vi "Write iterator.vi"(10 "iterator":refnum<data-value>, 11 "Circular Buffer in":refnum<class "Circular Buffer.lvclass">) -> (3 "Circular Buffer out":refnum<class "Circular Buffer.lvclass">)   [LabVIEW 2021, in "d20.lvlib" / "Circular Buffer.lvclass"]
uses:
  Circular Buffer.lvclass
  INode/INode.lvclass
  Circular Buffer.lvclass/Circular Buffer.ctl
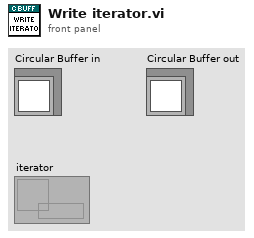
[diagram p1: front panel]
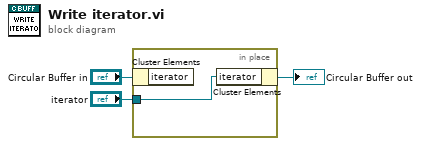
[diagram p0: block diagram]
diagram:
  n1 = in-place {
    in-place-border: "iterator" -> [w4]
    n2 = in-place-cluster #1("Circular Buffer in") -> ()  [unwired: 1 out]
    n3 = in-place-cluster #1("iterator"=w4) -> (→"Circular Buffer out":refnum<class "Circular Buffer.lvclass">)
  }
